vi "DAQ_Test.vi"() -> ()   [LabVIEW 2009]
uses:
  <userlib>/LV-LINK/OLCreateTask.vi
  <userlib>/LV-LINK/PolySubVIs/CreateAinChan.vi
  <userlib>/LV-LINK/PolySubVIs/OLReadSingle.vi
  <vilib>/ptbypt/NI_PtbyPt.lvlib
panel:
  in  "?":bool
  out "Acquired Data":dbl(graph)
  in  "Channels":string="Ain 0"
  # "Untimed Analog Input Using Single Value Input"
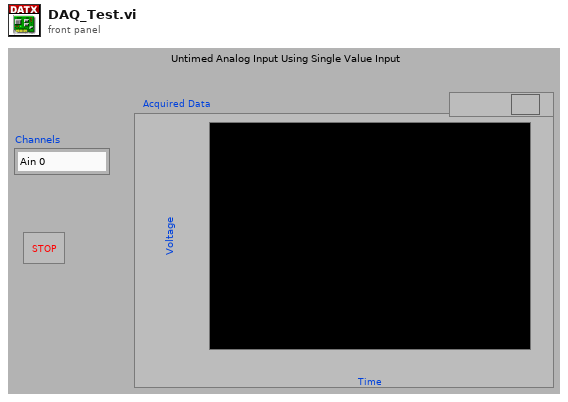
[diagram p1: front panel]
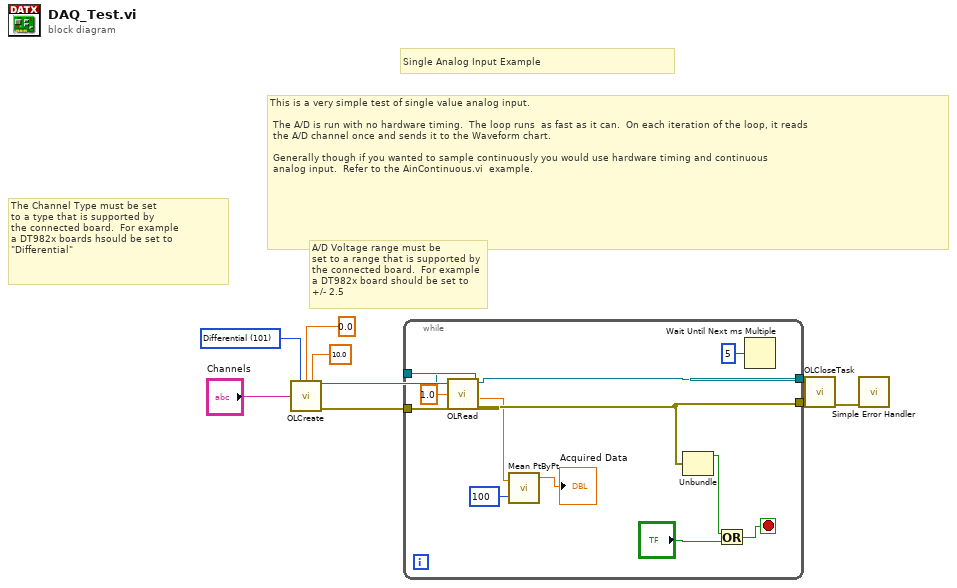
[diagram p0: block diagram]
diagram:
  w3 = 101 items=["SingleEnded"=100, "Differential"=101] ("Channel Type")
  # "The Channel Type must be set\nto a type that is supported by \nthe connected board.  For example\na DT982x boards hsould be set to\n\"Differential\""
  # "A/D Voltage range must be\nset to a range that is supported by \nthe connected board.  For example\na DT982x board should be set to \n+/- 2.5"
  # "Single Analog Input Example"
  # "This is a very simple test of single value analog input. \n\n The A/D is run with no hardware timing.  The loop runs  as fast as it can.  On each iteration of the loop, it reads\n the A/D channel once and sends it to the Waveform chart.\n\n Generally though if you wanted to sample continuously you would use hardware timing and continuous\n analog input.  Refer to the AinContinuous.vi  example."
  n1 = call-poly "OLCreate.vi"("Channel Type"=w3, "Range Min"=0.0, "Range Max"=10.0, "Channel"="Channels") -> ("Task Out"=w8:refnum<k24>, "error out"=w7:errorcluster)  [unwired: 10 in]
  n2 = while {
    tunnel: w8 -> [w21]
    tunnel: w7 -> [w20]
    tunnel: [w18] -> w6
    tunnel: [w17] -> w5
    stop <- w14 stop-if-true
    n3 = call-poly <userlib>:"OLRead.vi"("error in (no error)"=w20, "Timeout"=1.0 ("Samples Per Channel"), "Task In"=w21) -> ("error out"=w17:errorcluster, "Data Value"=w11:dbl, "Task Out"=w18:refnum<k24>)  [unwired: 6 in]
    n4 = call <vilib>:"Mean PtByPt.vi"("x"=w11, "sample length"=100) -> ("mean"=→"Acquired Data":dbl)  [unwired: 2 in, 1 out]
    n5 = Unbundle(w17) -> ("status"=w16:bool)  [unwired: 2 out]
    n6 = Or(x=w16, y="?") -> (x .or. y?=w14:bool)
    n7 = Wait Until Next ms Multiple(millisecond multiple=u32 5) -> ()  [unwired: 1 out]
  }
  n8 = call <userlib>:"OLCloseTask.vi"("Error in"=w5, "Task In"=w6) -> ("Error Out"=w4:errorcluster)  [unwired: 9 in]
  n9 = call <vilib>:"Simple Error Handler.vi"("error in (no error)"=w4) -> ()  [unwired: 4 in, 5 out]
